vi "Stepper_motor_move.vi"(0 "Arduino Error":errorcluster, 1 "X forward":bool, 2 "Step Size (mm)":sgl, 7 "X Back":bool, 9 "Y forward":bool, 12 "Y back":bool) -> (4 "error out":errorcluster)   [LabVIEW 2019]
uses:
  SiPM_Tests_Global_Var.vi
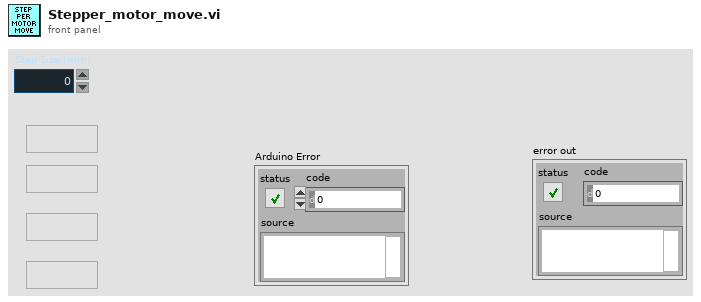
[diagram p1: front panel]
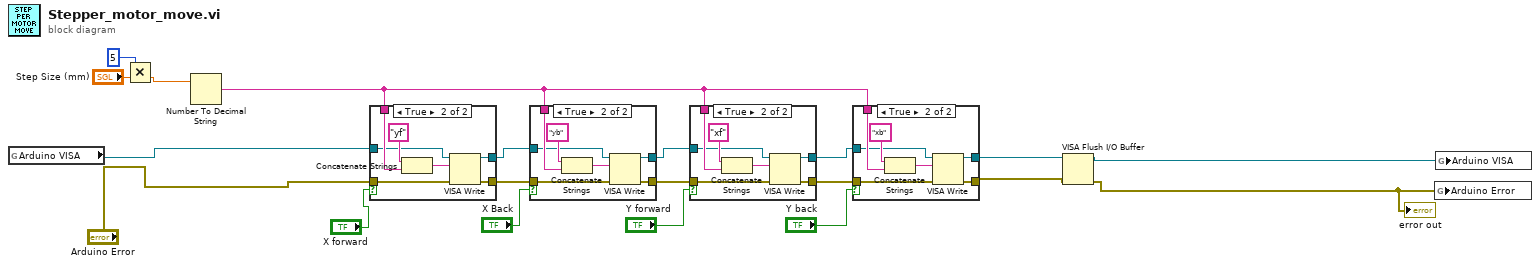
[diagram p0: block diagram]
diagram:
  n1 = global read "SiPM_Tests_Global_Var.vi" "Arduino VISA"() -> (w8:refnum<visa-resource-name>)
  n2 = Multiply(x=u32 5, y="Step Size (mm)") -> (x*y=w2:sgl)
  n3 = Number To Decimal String(number=w2) -> (decimal integer string=w20:string)  [unwired: 1 in]
  n4 = case shown="True" "X forward" {
    tunnel: w20 -> [_ w28]
    tunnel: w8 -> [w22 w26]
    tunnel: "Arduino Error" -> [w21 w25]
    tunnel: [w22 w24] -> w11
    tunnel: [w21 w23] -> w12
    frame False {
    }
    frame True {
      n5 = Concatenate Strings("yf" ("string"), w28) -> (w27:string)
      n6 = VISA Write(VISA resource name=w26, write buffer=w27, error in (no error)=w25) -> (VISA resource name out=w24:refnum<visa-resource-name>, error out=w23:errorcluster)  [unwired: 1 out]
    }
  }
  n7 = case shown="True" "X Back" {
    tunnel: w20 -> [_ w37]
    tunnel: w11 -> [w31 w35]
    tunnel: w12 -> [w30 w34]
    tunnel: [w31 w33] -> w16
    tunnel: [w30 w32] -> w15
    frame False {
    }
    frame True {
      n8 = Concatenate Strings("yb" ("string"), w37) -> (w36:string)
      n9 = VISA Write(VISA resource name=w35, write buffer=w36, error in (no error)=w34) -> (VISA resource name out=w33:refnum<visa-resource-name>, error out=w32:errorcluster)  [unwired: 1 out]
    }
  }
  n10 = case shown="True" "Y forward" {
    tunnel: w20 -> [_ w46]
    tunnel: w16 -> [w40 w44]
    tunnel: w15 -> [w39 w43]
    tunnel: [w40 w42] -> w19
    tunnel: [w39 w41] -> w18
    frame False {
    }
    frame True {
      n11 = Concatenate Strings("xf" ("string"), w46) -> (w45:string)
      n12 = VISA Write(VISA resource name=w44, write buffer=w45, error in (no error)=w43) -> (VISA resource name out=w42:refnum<visa-resource-name>, error out=w41:errorcluster)  [unwired: 1 out]
    }
  }
  n13 = case shown="True" "Y back" {
    tunnel: w20 -> [_ w55]
    tunnel: w19 -> [w49 w53]
    tunnel: w18 -> [w48 w52]
    tunnel: [w49 w51] -> w6
    tunnel: [w48 w50] -> w5
    frame False {
    }
    frame True {
      n14 = Concatenate Strings("xb" ("string"), w55) -> (w54:string)
      n15 = VISA Write(VISA resource name=w53, write buffer=w54, error in (no error)=w52) -> (VISA resource name out=w51:refnum<visa-resource-name>, error out=w50:errorcluster)  [unwired: 1 out]
    }
  }
  n16 = VISA Flush I/O Buffer(VISA resource name=w6, error in (no error)=w5) -> (VISA resource name out=w4:refnum<visa-resource-name>, error out=w3:errorcluster)  [unwired: 1 in]
  "error out" <- w3
  n17 = global write "SiPM_Tests_Global_Var.vi" "Arduino Error"(w3) -> ()
  n18 = global write "SiPM_Tests_Global_Var.vi" "Arduino VISA"(w4) -> ()
